vi "zadanie 1.vi"() -> ()   [LabVIEW 2013]
panel:
  out "Массив В":dbl[][](array[numeric])
  out "Массив А":dbl[][](array[numeric])
  out "Вывод":dbl[][](array[numeric])
  in  "Размер массива":dbl
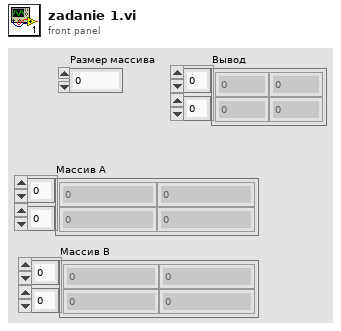
[diagram p1: front panel]
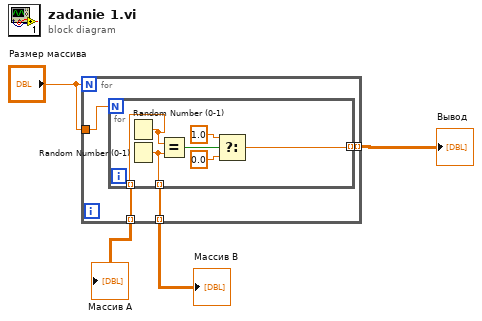
[diagram p0: block diagram]
diagram:
  n1 = for {
    N: "Размер массива" -> [_]
    tunnel: "Размер массива" -> [w5]
    tunnel: [w8] -> w3 mode=indexing
    tunnel: [w7] -> w2 mode=indexing
    tunnel: [w6] -> w1 mode=indexing
    n2 = for {
      N: w5 -> [_]
      tunnel: [w11] -> w8 mode=indexing
      tunnel: [w10] -> w7 mode=indexing
      tunnel: [w9] -> w6 mode=indexing
      n3 = Random Number (0-1)() -> (number: 0 to 1=w10:dbl)
      n4 = Random Number (0-1)() -> (number: 0 to 1=w9:dbl)
      n5 = Equal?(x=w10, y=w9) -> (x = y?=w12:bool)
      n6 = Select(t=1.0, s=w12, f=0.0) -> (s? t:f=w11:dbl)
    }
  }
  "Вывод" <- w3
  "Массив А" <- w2
  "Массив В" <- w1
